vi "Compare Topologies UI.vi"() -> ()   [LabVIEW 2017]
panel:
  in  "Modified Topology Path":path
  in  "Base Topology Path":path
  in  "Differences":i32(listbox)
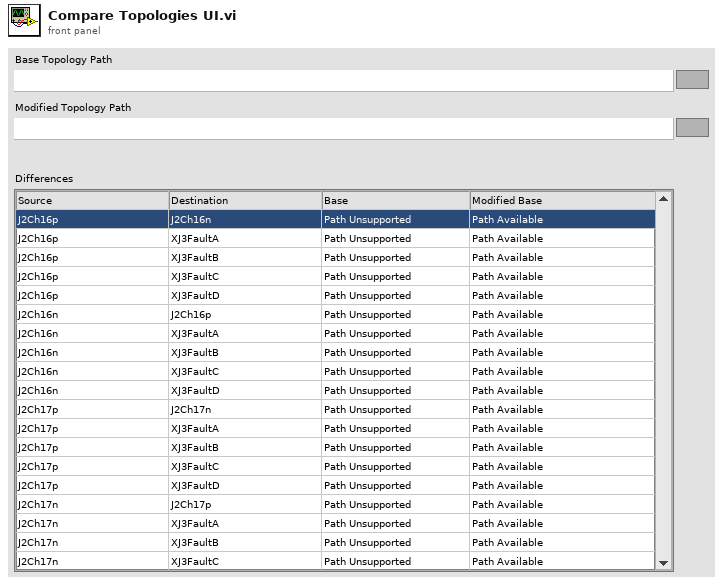
[diagram p1: front panel]
types:
  T1 = typedef "SLSC Switch.lvlib/Path Capability.ctl" = i32
  T2 = cluster{string, string, "path capability":T1, "path capability":T1}[]
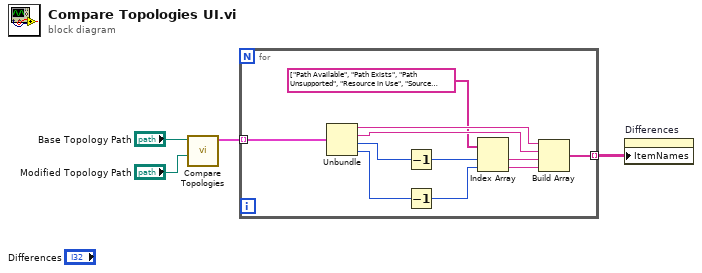
[diagram p0: block diagram]
diagram:
  n1 = call "Compare Topologies.vi"("Modified Base Topology"="Modified Topology Path", "Base Topology"="Base Topology Path") -> ("Differences"=w2:T2)  [unwired: 8 in, 1 out]
  n2 = for {
    tunnel: w2 -> [w15] mode=indexing
    tunnel: [w12] -> w1 mode=indexing
    n3 = Unbundle(w15) -> (w14:string, w13:string, "path capability"=w10:T1, "path capability"=w9:T1)
    n4 = Decrement(x=w10) -> (x-1=w6:T1)
    n5 = Decrement(x=w9) -> (x-1=w5:T1)
    n6 = Index Array(array=string[] ["Path Available", "Path Exists", "Path Unsupported", "Resource in Use", "Source Conflict", "Channel Not Available"] ("Strings []"), index #1=w6, index #2=w5) -> (element #1=w8:string, element #2=w7:string)
    n7 = Build Array(w14, w13, w8, w7) -> (w12:string[])
  }
  n8 = property on="Differences" class="MCListbox (strict)"("ItemNames"=w1) -> ()  [unwired: 2 in, 2 out]
